vi "Do.vi"(8 "error in (no error)":errorcluster, 10 "Actor in":refnum<class "Actor.lvclass">, 11 "Batch Message":refnum<class "Batch Msg.lvclass">) -> (0 "error out":errorcluster, 2 "Actor out":refnum<class "Actor.lvclass">)   [LabVIEW 2017, in "AF_Messages-PPL.lvlib" / "Batch Msg.lvclass"]
uses:
  Batch Msg.lvclass
  PPLs/Actor Framework.lvlibp/Actor/Actor.lvclass
  Batch Msg.lvclass/Batch Msg.ctl
  PPLs/Actor Framework.lvlibp/Message/Message.lvclass
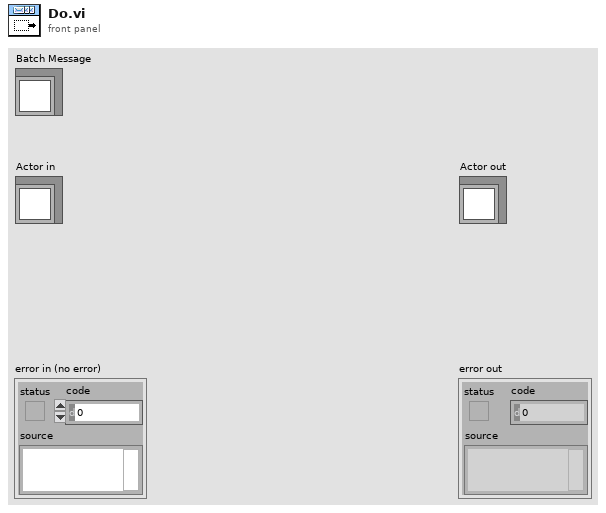
[diagram p1: front panel]
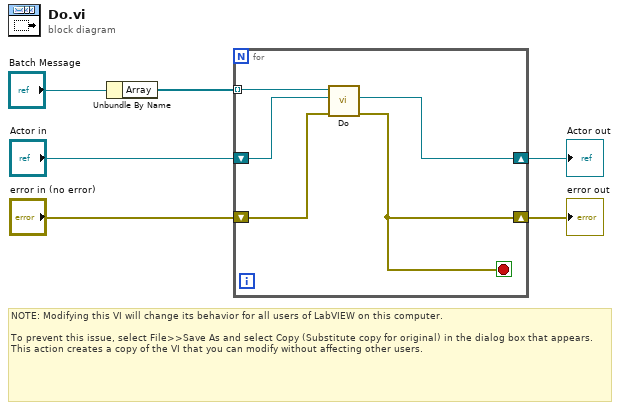
[diagram p0: block diagram]
diagram:
  # "NOTE: Modifying this VI will change its behavior for all users of LabVIEW on this computer.\n\nTo prevent this issue, select File>>Save As and select Copy (Substitute copy for original) in the dialog box that appears. This action creates a copy of the VI that you can modify without affecting other users."
  n1 = Unbundle By Name("Batch Message") -> ("Array"=w5:refnum<class "Message.lvclass">[])
  n2 = for {
    tunnel: w5 -> [w11] mode=indexing
    shift-right: [w9] -> w3
    shift-left: "Actor in" -> [w10]
    shift-right: [w7] -> w1
    shift-left: "error in (no error)" -> [w8]
    stop <- w7 stop-if-true
    n3 = call-dynamic "Do.vi"("error in (no error)"=w8, "Actor in"=w10, "Message"=w11) -> ("error out"=w7:errorcluster, "Actor out"=w9:refnum<class "Actor.lvclass">)  [unwired: 7 in]
  }
  "error out" <- w1
  "Actor out" <- w3
